vi "CurrentServoStatus.vi"(2 "New Servo Status":cluster{"mode":string, "position":dbl} {"position" min=0.0 max=180.0 step=1.0}, 3 "Operation":enum16{"Get", "Set"}(ring)) -> (1 "Current Servo Status":cluster{"mode":string, "position":dbl} {"position" min=0.0 max=180.0 step=1.0})   [LabVIEW 2024]
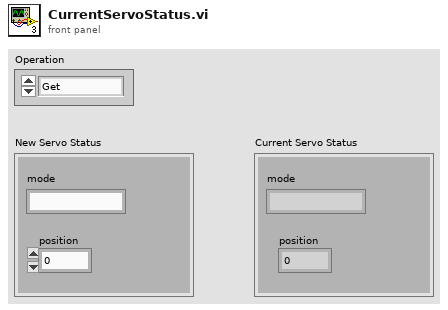
[diagram p1: front panel]
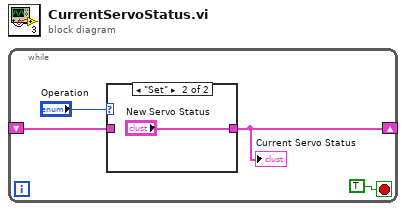
[diagram p0: block diagram]
diagram:
  n1 = while {
    shift-right: [w1] -> _
    shift-left: _ -> [w2]
    stop <- TRUE stop-if-true
    n2 = case shown="\"Set\"" "Operation" {
      tunnel: w2 -> [w5 _]
      tunnel: [w5 "New Servo Status"] -> w1
      frame "Get", Default {
      }
      frame "Set" {
      }
    }
    "Current Servo Status" <- w1
  }
